vi "Shoot Until No Balls_wrapper.vi"() -> ()   [LabVIEW 2019]
uses:
  <vilib>/Rock Robotics/WPI/Framework/Command Status Info.ctl
  <vilib>/Rock Robotics/WPI/Framework/Completion Status.ctl
  <vilib>/Rock Robotics/WPI/Framework/Completion Notifier.ctl
panel:
  in  "Flywheel Value":dbl
  in  "Turret Value":dbl
  in  "Auto-Align":bool
  in  "Hood Value":dbl
  out "Command Info Out":T1
  in  "Command Info In":T1
  in  "Description":string
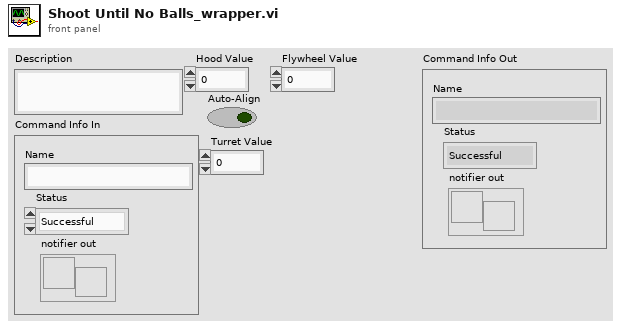
[diagram p1: front panel]
types:
  T1 = typedef "Command Status Info.ctl" = cluster{"Name":string, "Status":T2, "notifier out":T3}
  T2 = typedef "Completion Status.ctl" = enum16{"Successful", "Aborted", "Incomplete"}
  T3 = typedef "Completion Notifier.ctl" = refnum<notifier>
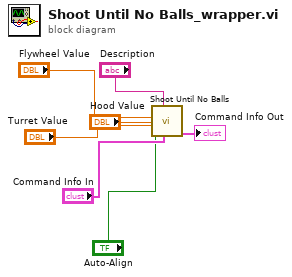
[diagram p0: block diagram]
diagram:
  n1 = call "Shoot Until No Balls.vi"("Command Info In"="Command Info In", "Description"="Description", "Auto-Align"="Auto-Align", "Turret Value"="Turret Value", "Flywheel Value"="Flywheel Value", "Hood Value"="Hood Value") -> ("Command Info Out"=→"Command Info Out":T1)  [unwired: 5 in]
